vi "GetHeader.vi"(8 "error in (no error)":errorcluster, 10 "Name":string, 11 "Headers In":variant) -> (0 "error out":errorcluster, 1 "Found?":bool, 2 "Data":string, 3 "Headers Out":variant)   [LabVIEW 2018]
doc: "Retrieves a named header from the received HTTP handshaking data.\nWebSockets API 1.3.0.13\nSam Sharp - Intelligent Energy\nCopyright (c) 2015, Intelligent Energy"
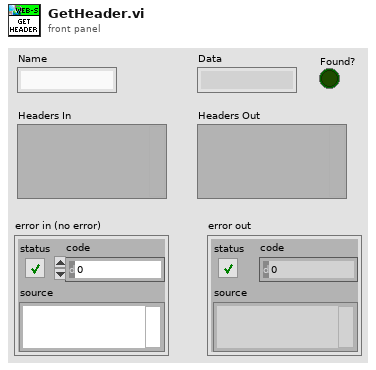
[diagram p1: front panel]
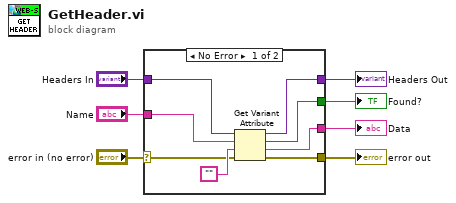
[diagram p0: block diagram]
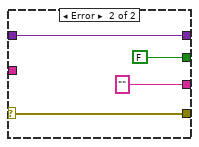
[diagram p2: hidden frame]
diagram:
  n1 = case shown="No Error" "error in (no error)" {
    selector: "error in (no error)" -> [w10 w19]
    tunnel: [w15 ""] -> w7
    tunnel: "Name" -> [w13 _]
    tunnel: "Headers In" -> [w12 w18]
    tunnel: [w11 w18] -> w4
    tunnel: [w9 w19] -> w2
    tunnel: [w8 FALSE] -> w1
    frame No Error {
      n2 = Get Variant Attribute(Variant=w12, name=w13, default value (empty Variant)="", error in=w10) -> (duplicate Variant=w11:variant, found=w8:bool, value=w15:string, error out=w9:errorcluster)
    }
    frame Error {
    }
  }
  "Data" <- w7
  "Headers Out" <- w4
  "error out" <- w2
  "Found?" <- w1
